vi "MP711134-12V.vi"(8 "error in (no error)":errorcluster) -> (0 "error in (out)":errorcluster)   [LabVIEW 2024, in "Multicom_MP711134-12V.lvlib"]
doc: "This template is for the Queued Message Handler design pattern.\n\nThe Event Handling Loop generates messages based on user interface actions.\n\nThe Message Handling Loop processes messages generated by the Event Handling Loop, or by other messages. The messages are string values, so new messages can be added easily to the Message Cases case structure in the Message Handling Loop. Each message cluster can also provide an optional value for Message Data, which is a variant that can be converted to whatever message-specific data is required."
uses:
  Multicom_MP711134-12V.lvlib
  controls/72-13360 UI Data.ctl
  PrivateControls/FGV_Queue_Control.ctl
  <vilib>/Instr/_visa.llb/VISA Configure Serial Port (Instr).vi
  <vilib>/Utility/error.llb/Error Cluster From Error Code.vi
  <vilib>/ErrorRing/Error Ring.xnode
  support/Message Queue/72-13360 Message Queue.lvlib
  support/User Event - Stop/72-13360 User Event - Stop.lvlib
  Launcher/Launcher_DTU.lvlib
panel:
  in  "Config":string
  in  "DUT":string
  out "RESISTANCE":string
  out "CURRENT":string
  out "VOLTAGE":string
  in  "VISA resource name":refnum<visa-resource-name>
  in  "SET_Current":dbl format="%#_4f"
  in  "SET_Voltage":dbl format="%#_4f"
  in  "Read_Res":bool
  in  "Read_Current":bool
  in  "Read_Voltage":bool
  in  "Set Current":bool
  out "Connected?":bool
  out "queue name 2":string
  out "queue name":string
  out "Display <Replace Me>":string
  in  "Output":bool
  in  "Set Voltage":bool
  in  "Exit":bool
  # "These controls have associated \"Value Changed\" events configured in the Event Structure on the diagram.\n\nReplace them (and reconfigure the Event Structure) with the controls you need for your application."
  # "This template is for the Queued Message Handler design pattern.\n\nSee the block diagram for more information on how to use this template."
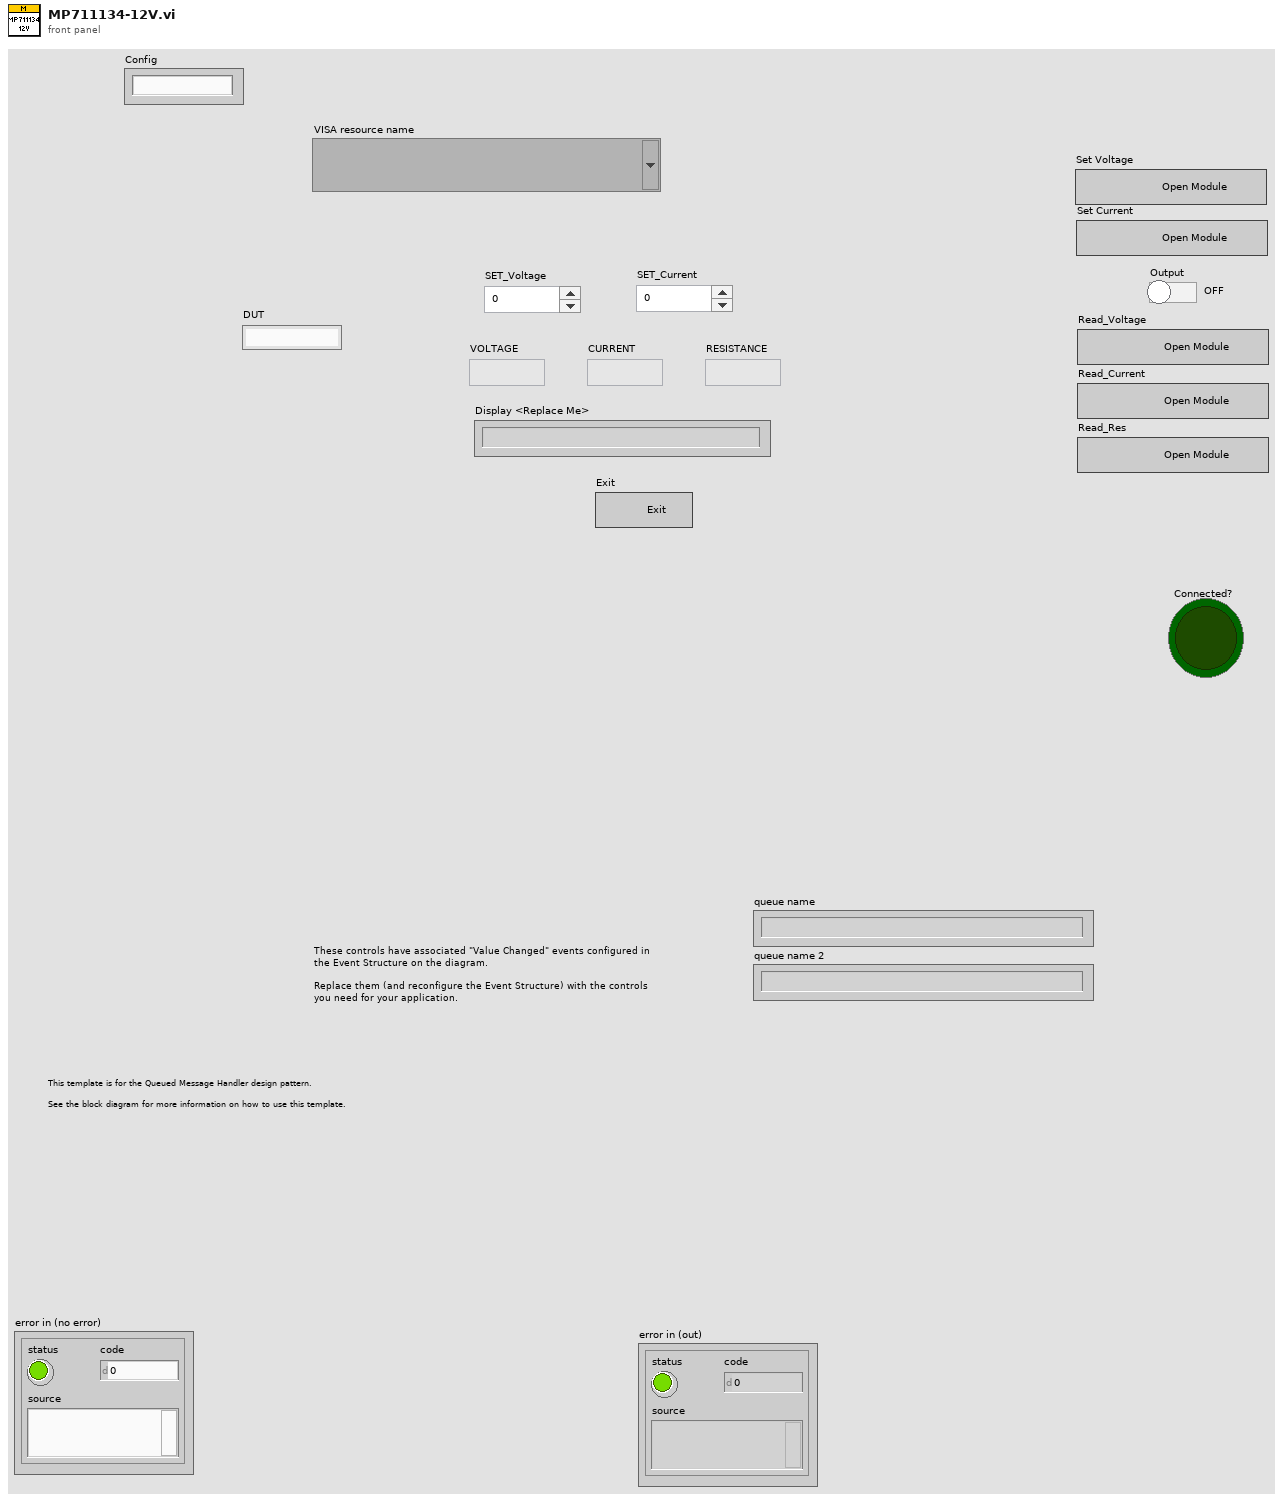
[diagram p1: front panel]
types:
  T1 = typedef "Multicom_MP711134-12V.lvlib/72-13360 UI Data.ctl" = cluster{"Boolean <Replace Me>":bool, "DUT":string, "Numeric <Replace Me>":dbl, "VISA":refnum<visa-resource-name>, "13360_Q":refnum<queue>, "notifier out":refnum<notifier>, "Config":string}
  T2 = typedef "Multicom_MP711134-12V.lvlib/FGV_Queue_Control.ctl" = enum16{"Release", "Get", "Set"}
  T3 = typedef "Multicom_MP711134-12V.lvlib/72-13360 Message Queue.lvlib/All Message Queues.ctl" = cluster{"UI":refnum<queue>, "QSM":refnum<queue>}
  T4 = cluster{"Message":string, "Message Data":variant}
  T5 = enum16{"Read", "Write", "All_sections", "All_values", "Remove key&section"}
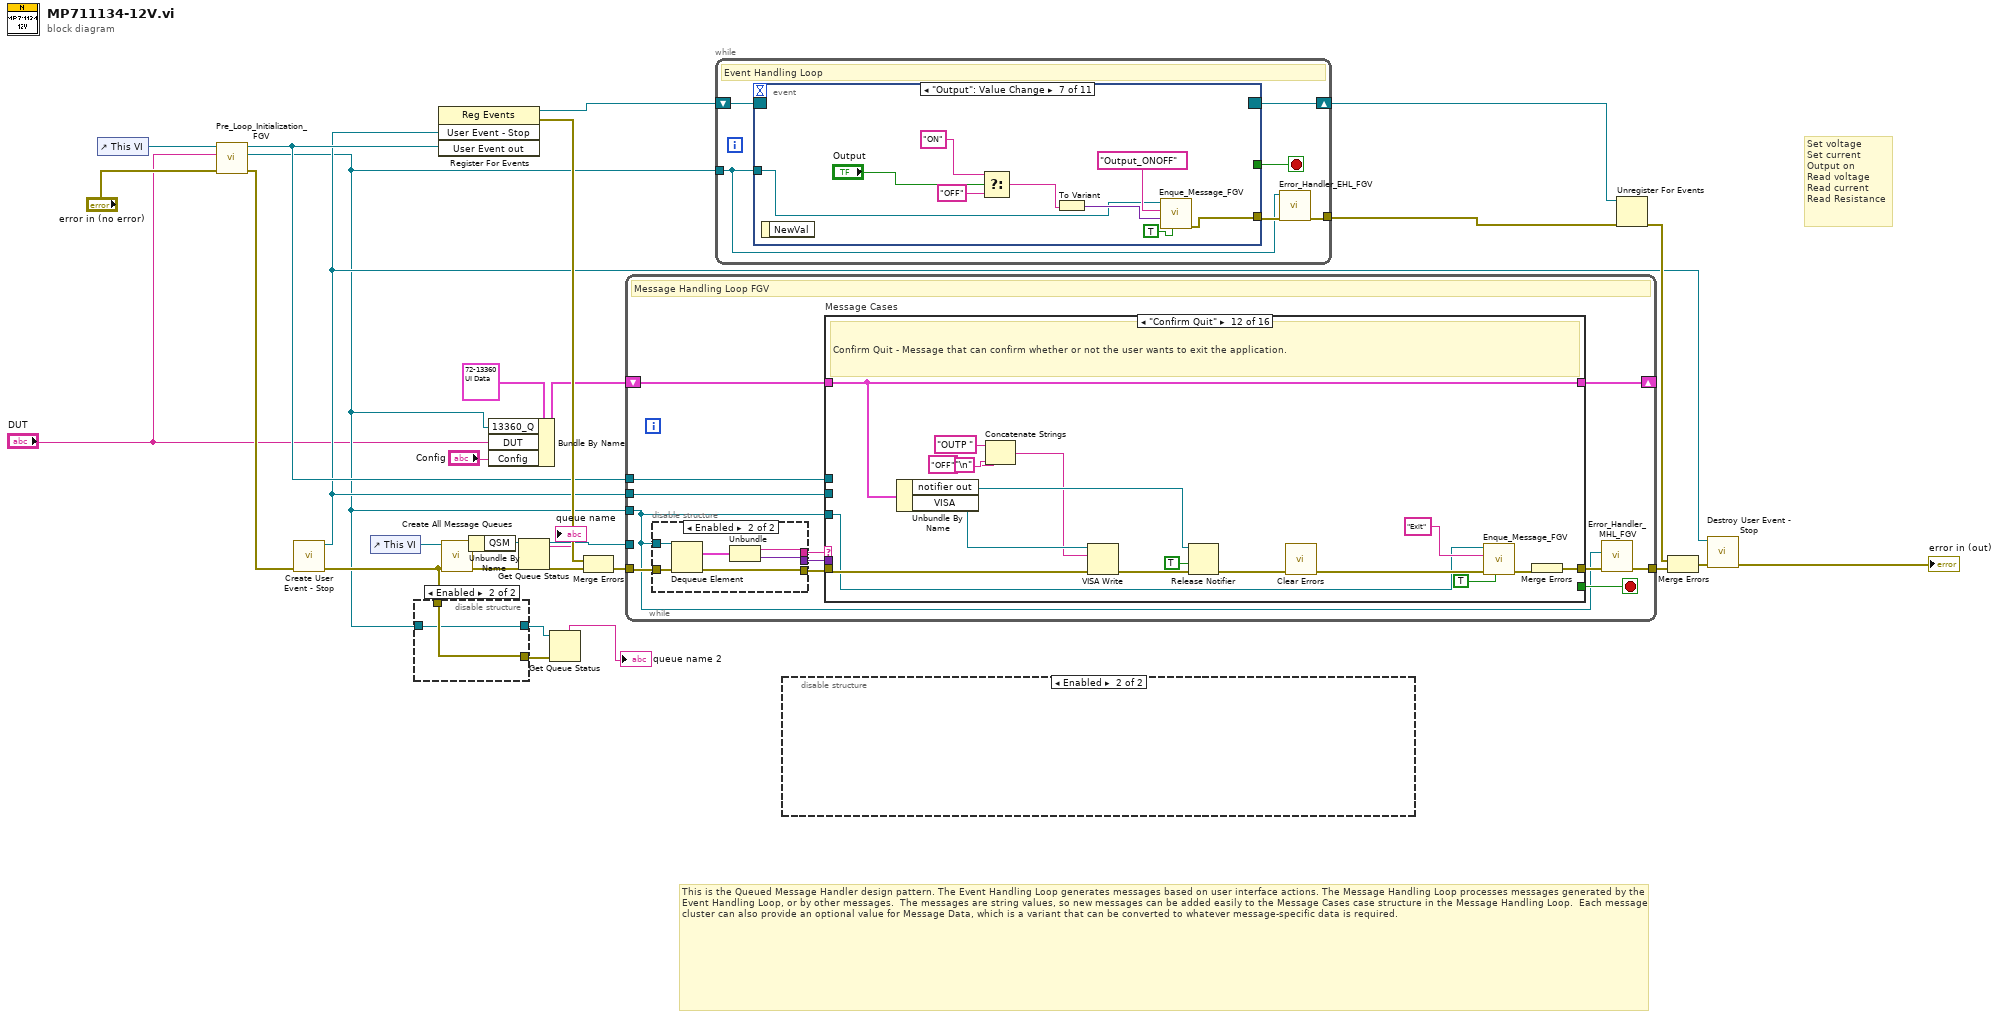
[diagram p0: block diagram]
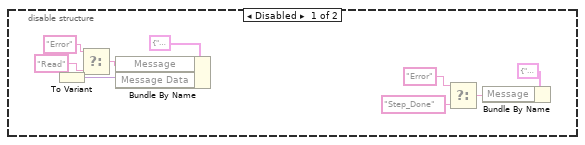
[diagram p2: hidden frame]
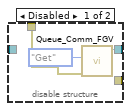
[diagram p3: hidden frame]
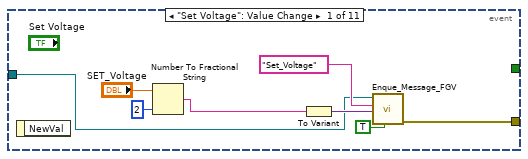
[diagram p4: hidden frame]
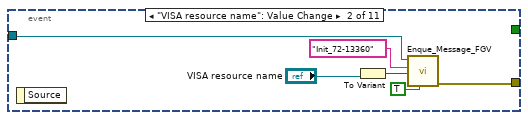
[diagram p5: hidden frame]
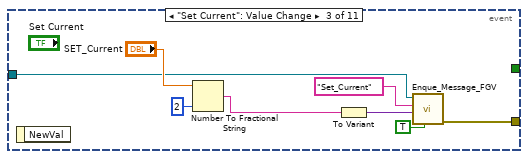
[diagram p6: hidden frame]
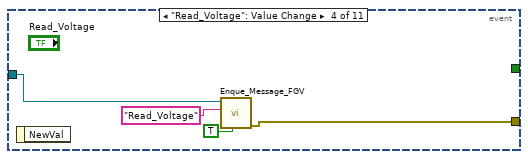
[diagram p7: hidden frame]
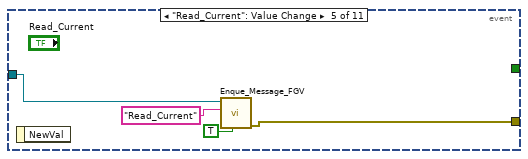
[diagram p8: hidden frame]
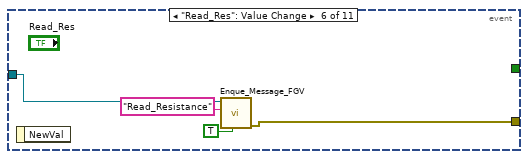
[diagram p9: hidden frame]
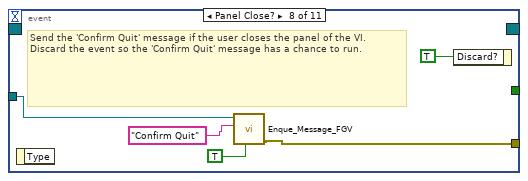
[diagram p10: hidden frame]
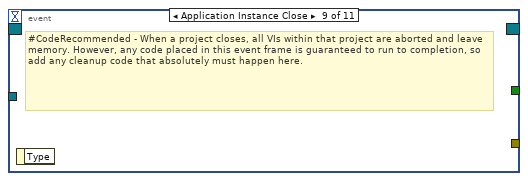
[diagram p11: hidden frame]
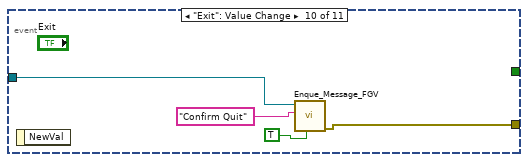
[diagram p12: hidden frame]
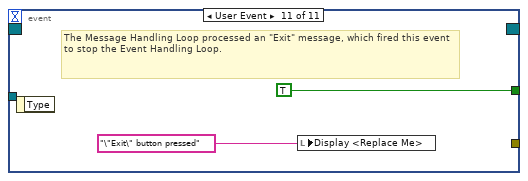
[diagram p13: hidden frame]
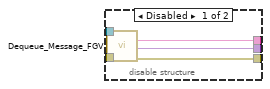
[diagram p14: hidden frame]
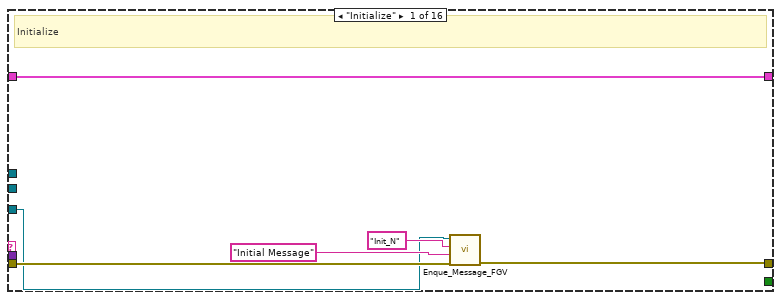
[diagram p15: hidden frame]
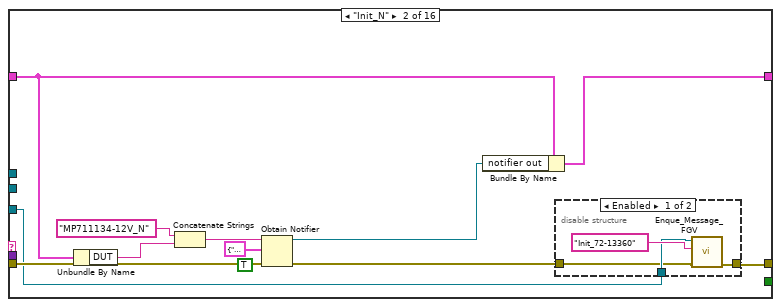
[diagram p16: hidden frame]
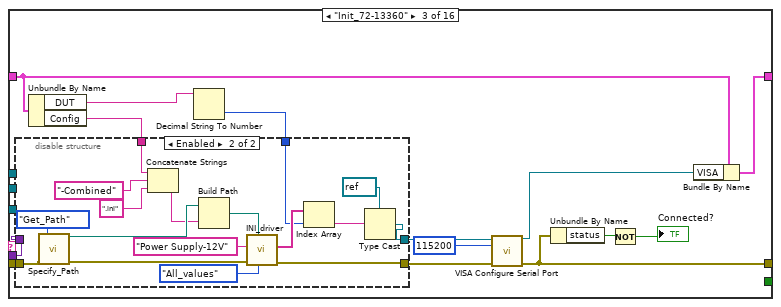
[diagram p18: hidden frame]
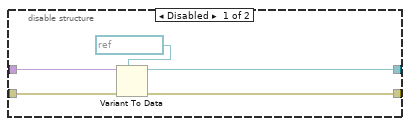
[diagram p19: hidden frame]
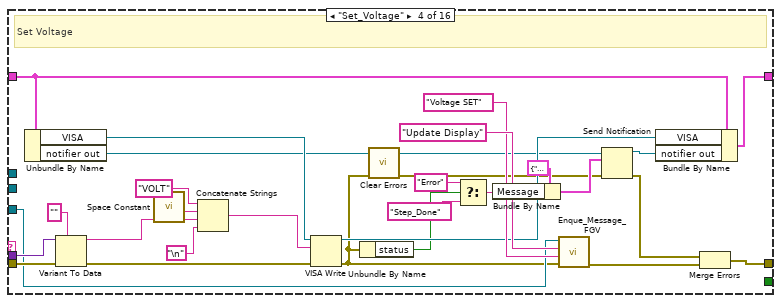
[diagram p20: hidden frame]
diagram:
  # "Set voltage\nSet current\nOutput on\nRead voltage \nRead current\nRead Resistance"
  # "This is the Queued Message Handler design pattern. The Event Handling Loop generates messages based on user interface actions. The Message Handling Loop processes messages generated by the Event Handling Loop, or by other messages.  The messages are string values, so new messages can be added easily to the Message Cases case structure in the Message Handling Loop.  Each message cluster can also provide an optional value for Message Data, which is a variant that can be converted to whatever message-specific data is required."
  n1 = control-ref of="This VI"() -> (w17:refnum<vi>)
  n2 = call "Pre_Loop_Initialization_FGV.vi"("error in (no error)"="error in (no error)", "DUT"="DUT", "VI in"=w17) -> ("error out"=w15:errorcluster, "queue out"=w3:refnum<queue>, "User Event out"=w7:refnum<user-event>)  [unwired: 6 in]
  n3 = call "Create User Event - Stop.vi"("error in (no error)"=w15) -> ("error out"=w10:errorcluster, "User Event - Stop"=w6:refnum<user-event>)  [unwired: 9 in]
  n4 = control-ref of="This VI"() -> (w13:refnum<vi>)
  n5 = disable-structure shown="Enabled" {
    disable-tunnel: w10 -> [w32 w34]
    disable-tunnel: [w30 w33] -> w9
    disable-tunnel: [_ w34] -> w5
    disable-tunnel: w3 -> [_ w33]
    frame Disabled {
      n6 = call "Queue_Comm_FGV.vi"("error in (no error)"=w32, "Enum"=FGV_Queue_Control."Get") -> ("queue Out"=w30:refnum<queue>)  [unwired: 8 in, 1 out]
    }
    frame Enabled {
    }
  }
  n7 = register-events(w6, w7) -> (reference out=w20:refnum<event-registration>, error out=w18:errorcluster)  [unwired: 2 in]
  n8 = call "Create All Message Queues.vi"("error in (no error)"=w10, "This VI"=w13) -> ("error out"=w29:errorcluster, "Message Queues out"=w28:T3)  [unwired: 8 in]
  n9 = Unbundle By Name(w28) -> ("QSM"=w26:refnum<queue>)
  n10 = Bundle By Name(cluster=T1 {"Boolean <Replace Me>"=FALSE, "DUT"="", "Numeric <Replace Me>"=0.0, "VISA"="", "13360_Q"=refnum, "notifier out"=refnum, "Config"=""} ("Data Cluster"), "13360_Q"=w3, "DUT"="DUT", "Config"="Config") -> (w4:T1)
  n11 = Get Queue Status(queue=w26) -> (queue out=w12:refnum<queue>, queue name=→"queue name":string)  [unwired: 2 in, 6 out]
  n12 = Get Queue Status(queue=w9, error in (no error)=w5) -> (queue name=→"queue name 2":string)  [unwired: 1 in, 7 out]
  n13 = Merge Errors(w18, w29) -> (w19:errorcluster)
  n14 = while {
    tunnel: w12 -> [_]
    shift-right: [w45] -> _
    shift-left: w4 -> [w46]
    tunnel: w7 -> [w43]
    tunnel: w19 -> [w42]
    tunnel: [w37] -> w27
    tunnel: w6 -> [w36]
    tunnel: w3 -> [w35]
    stop <- w44 stop-if-true
    # "Message Handling Loop FGV"
    n15 = disable-structure shown="Enabled" {
      disable-tunnel: w42 -> [w50 w56]
      disable-tunnel: [w49 w54] -> w41
      disable-tunnel: [w48 w51] -> w40
      disable-tunnel: [w47 w52] -> w39
      disable-tunnel: w35 -> [_ w55]
      frame Disabled {
        n16 = call "Dequeue_Message_FGV.vi"("error in (no error)"=w50) -> ("error out"=w49:errorcluster, "Message Data"=w48:variant, "Message"=w47:string)  [unwired: 8 in]
      }
      frame Enabled {
        n17 = Dequeue Element(queue=w55, error in (no error)=w56) -> (element=w53:T4, error out=w54:errorcluster)  [unwired: 1 in, 2 out]
        n18 = Unbundle(w53) -> ("Message"=w52:string, "Message Data"=w51:variant)
      }
    }
    n19 = case "Message Cases" shown="\"Confirm Quit\"" w39 {
      selector: w39 -> [_ _ _ _ _ _ _ _ _ _ _ _ _ _ _ w340]
      tunnel: w41 -> [w58 w74 w93 w140 w157 w200 w235 w243 w274 w281 w291 w306 w317 w320 w331 _]
      tunnel: [w61 w63 w89 w144 w169 w183 w218 w242 w258 w282 w285 w308 w314 w318 w321 w341] -> w38
      tunnel: w46 -> [w62 w72 w83 w136 w159 w198 w233 w246 w270 w283 w290 w303 w316 w319 w326 w342]
      tunnel: [w62 w67 w92 w134 w159 w196 w231 w246 w264 w283 w290 w303 w316 w319 w326 w342] -> w45
      tunnel: [_ _ _ _ _ _ _ _ _ _ _ _ _ _ TRUE _] -> w44
      tunnel: w40 -> [_ _ w85 w138 w161 _ _ _ w267 w280 w289 _ _ _ w333 _]
      tunnel: w43 -> [_ _ _ _ _ _ _ _ _ _ _ _ _ _ w334 _]
      tunnel: w36 -> [_ _ _ _ _ _ _ _ _ _ _ _ _ _ w329 _]
      tunnel: w35 -> [w57 w65 _ w128 w155 w184 w219 w241 w259 _ _ w299 _ _ w322 _]
      frame "Initialize" {
        # "Initialize"
        n20 = call "Enque_Message_FGV.vi"("error in (no error)"=w58, "Message Data"="Initial Message" ("Initial Message"), "Message"="Init_N", "queue in"=w57) -> ("error out"=w61:errorcluster)  [unwired: 7 in]
      }
      frame "Init_N" {
        n21 = Unbundle By Name(w72) -> ("DUT"=w71:string)
        n22 = Concatenate Strings("MP711134-12V_N", w71) -> (w70:string)
        n23 = Obtain Notifier(name (unnamed)=w70, notification data type=T4 {"Message"="", "Message Data"=variant} ("notification"), create if not found? (T)=TRUE, error in (no error)=w74) -> (notifier out=w66:refnum<notifier>, error out=w64:errorcluster)  [unwired: 1 out]
        n24 = Bundle By Name(cluster=w72, "notifier out"=w66) -> (w67:T1)
        n25 = disable-structure shown="Enabled" {
          disable-tunnel: w65 -> [w77 _]
          disable-tunnel: w64 -> [w76 w79]
          disable-tunnel: [w75 w79] -> w63
          frame Enabled {
            n26 = call "Enque_Message_FGV.vi"("error in (no error)"=w76, "Message"="Init_72-13360", "queue in"=w77) -> ("error out"=w75:errorcluster)  [unwired: 8 in]
          }
          frame Disabled {
          }
        }
      }
      frame "Init_72-13360" {
        n27 = Unbundle By Name(w83) -> ("DUT"=w81:string, "Config"=w82:string)
        n28 = Decimal String To Number(string=w81) -> (number=w80:i32)  [unwired: 2 in, 1 out]
        n29 = disable-structure shown="Enabled" {
          disable-tunnel: w93 -> [w98 w103]
          disable-tunnel: [w97 w101] -> w86
          disable-tunnel: w85 -> [w96 _]
          disable-tunnel: [w94 w102] -> w84
          disable-tunnel: w82 -> [_ w100]
          disable-tunnel: w80 -> [_ w99]
          frame Disabled {
            n30 = Variant To Data(error in=w98, type=refnum<visa-resource-name> "COM27" ("VISA resource name"), Variant=w96) -> (data=w94:refnum<visa-resource-name>, error out=w97:errorcluster)
          }
          frame Enabled {
            n31 = call "Specify_Path.vi"("Path_Enum"=enum16{"Find_Path", "Get_Path"}."Get_Path", "error in (no error)"=w103) -> ("Configurations"=w112:path, "error out"=w108:errorcluster)  [unwired: 6 in, 6 out]
            n32 = Concatenate Strings(w100, "-Combined" ("string"), ".ini" ("string")) -> (w111:string)
            n33 = Build Path(base path=w112, name or relative path=w111) -> (appended path=w110:path)
            n34 = call "INI_driver.vi"("Enum"=T5."All_values", "instrument file path"=w110, "error in (no error)"=w108, "Section"="Power Supply-12V") -> ("error out"=w101:errorcluster, "Values out"=w106:string[])  [unwired: 4 in, 2 out]
            n35 = Index Array(array=w106, index=w99) -> (element=w105:string)
            n36 = Type Cast(type=refnum<visa-resource-name> refnum ("VISA resource name"), x=w105) -> (*(type *) &x=w102:refnum<visa-resource-name>)
          }
        }
        n37 = call-poly "VISA Configure Serial Port"("VISA resource name"=w84, "baud rate (9600)"=u32 115200, "error in (no error)"=w86) -> ("VISA resource name out"=w90:refnum<visa-resource-name>, "error out"=w89:errorcluster)  [unwired: 11 in]
        n38 = Unbundle By Name(w89) -> ("status"=w88:bool)
        n39 = Not(x=w88) -> (.not. x?=→"Connected?":bool)
        n40 = Bundle By Name(cluster=w83, "VISA"=w90) -> (w92:T1)
      }
      frame "Set_Voltage" {
        # "Set Voltage"
        n41 = Unbundle By Name(w136) -> ("VISA"=w129:refnum<visa-resource-name>, "notifier out"=w122:refnum<notifier>)
        n42 = Variant To Data(error in=w140, type="", Variant=w138) -> (data=w131:string, error out=w139:errorcluster)
        n43 = call <vilib>:"Space Constant.vi"() -> ("String"=w116:string)
        n44 = Concatenate Strings("VOLT", w116, w131, "\n") -> (w132:string)
        n45 = VISA Write(VISA resource name=w129, write buffer=w132, error in (no error)=w139) -> (VISA resource name out=w133:refnum<visa-resource-name>, error out=w118:errorcluster)  [unwired: 1 out]
        n46 = Unbundle By Name(w118) -> ("status"=w117:bool)
        n47 = call <vilib>:"Clear Errors.vi"("error in (no error)"=w118) -> ("error out"=w119:errorcluster)  [unwired: 5 in, 1 out]
        n48 = Select(t="Error" ("f"), s=w117, f="Step_Done" ("Message")) -> (s? t:f=w125:string)
        n49 = Bundle By Name(cluster=T4 {"Message"="", "Message Data"=variant} ("notification"), "Message"=w125) -> (w121:T4)
        n50 = call "Enque_Message_FGV.vi"("error in (no error)"=w118, "Message Data"="Voltage SET" ("\"Do Something\" button pressed"), "Message"="Update Display", "queue in"=w128) -> ("error out"=w143:errorcluster)  [unwired: 7 in]
        n51 = Send Notification(notification=w121, notifier=w122, error in (no error)=w119) -> (notifier out=w123:refnum<notifier>, error out=w120:errorcluster)
        n52 = Bundle By Name(cluster=w136, "VISA"=w133, "notifier out"=w123) -> (w134:T1)
        n53 = Merge Errors(w120, w143) -> (w144:errorcluster)
      }
      frame "Set_Current" {
        # "Set current"
        n54 = Unbundle By Name(w159) -> ("notifier out"=w154:refnum<notifier>, "VISA"=w156:refnum<visa-resource-name>)
        n55 = Variant To Data(type="", Variant=w161) -> (data=w160:string)  [unwired: 1 in, 1 out]
        n56 = call <vilib>:"Space Constant.vi"() -> ("String"=w162:string)
        n57 = Concatenate Strings("CURR", w162, w160, "\n") -> (w163:string)
        n58 = VISA Write(VISA resource name=w156, write buffer=w163, error in (no error)=w157) -> (error out=w146:errorcluster)  [unwired: 2 out]
        n59 = Unbundle By Name(w146) -> ("status"=w145:bool)
        n60 = Select(t="Error" ("f"), s=w145, f="Step_Done" ("Message")) -> (s? t:f=w149:string)
        n61 = call <vilib>:"Clear Errors.vi"("error in (no error)"=w146) -> ("error out"=w153:errorcluster)  [unwired: 5 in, 1 out]
        n62 = Bundle By Name(cluster=T4 {"Message"="", "Message Data"=variant} ("notification"), "Message"=w149) -> (w147:T4)
        n63 = Send Notification(notification=w147, notifier=w154, error in (no error)=w153) -> (error out=w152:errorcluster)  [unwired: 1 out]
        n64 = call "Enque_Message_FGV.vi"("error in (no error)"=w146, "Message Data"="CURRENT SET" ("\"Do Something\" button pressed"), "Message"="Update Display", "queue in"=w155) -> ("error out"=w168:errorcluster)  [unwired: 7 in]
        n65 = Merge Errors(w152, w168) -> (w169:errorcluster)
      }
      frame "Read_Voltage" {
        # "Read Voltage"
        n66 = Unbundle By Name(w198) -> ("notifier out"=w181:refnum<notifier>, "VISA"=w197:refnum<visa-resource-name>)
        n67 = Concatenate Strings("MEAS:VOLT?", "\n") -> (w185:string)
        n68 = VISA Write(VISA resource name=w197, write buffer=w185, error in (no error)=w200) -> (VISA resource name out=w193:refnum<visa-resource-name>, error out=w194:errorcluster)  [unwired: 1 out]
        n69 = flat-sequence {
          tunnel: w194 -> [w205]
          tunnel: [w205] -> w188
          tunnel: w193 -> [w204]
          tunnel: [w204] -> w189
          frame #0 {
            n70 = Wait (ms)(milliseconds to wait=u32 500) -> ()  [unwired: 1 out]
          }
        }
        n71 = property class="Instr"(reference=w189, error in=w188) -> (reference out=w192:refnum<visa-resource-name>, error out=w191:errorcluster, "Bytes at Port"=w190:u32)
        n72 = VISA Read(VISA resource name=w192, byte count=w190, error in (no error)=w191) -> (VISA resource name out=w195:refnum<visa-resource-name>, read buffer=w174:string, error out=w172:errorcluster)  [unwired: 1 out]
        "VOLTAGE" <- w174
        n73 = To Variant(anything=w174) -> (Variant=w177:variant)
        n74 = Unbundle By Name(w172) -> ("status"=w171:bool)
        n75 = Select(t="Error" ("f"), s=w171, f="Read" ("Message")) -> (s? t:f=w180:string)
        n76 = Bundle By Name(cluster=T4 {"Message"="", "Message Data"=variant} ("notification"), "Message"=w180, "Message Data"=w177) -> (w175:T4)
        n77 = call <vilib>:"Clear Errors.vi"("error in (no error)"=w172) -> ("error out"=w173:errorcluster)  [unwired: 5 in, 1 out]
        n78 = Send Notification(notification=w175, notifier=w181, error in (no error)=w173) -> (notifier out=w182:refnum<notifier>, error out=w170:errorcluster)
        n79 = Bundle By Name(cluster=w198, "VISA"=w195, "notifier out"=w182) -> (w196:T1)
        n80 = call "Enque_Message_FGV.vi"("error in (no error)"=w172, "Message Data"="Read Voltage" ("\"Do Something\" button pressed"), "Message"="Update Display", "queue in"=w184) -> ("error out"=w199:errorcluster)  [unwired: 7 in]
        n81 = Merge Errors(w170, w199) -> (w183:errorcluster)
      }
      frame "Read_Current" {
        # "Read Voltage"
        n82 = Unbundle By Name(w233) -> ("notifier out"=w206:refnum<notifier>, "VISA"=w232:refnum<visa-resource-name>)
        n83 = Concatenate Strings("MEAS:CURR?", "\n") -> (w220:string)
        n84 = VISA Write(VISA resource name=w232, write buffer=w220, error in (no error)=w235) -> (VISA resource name out=w228:refnum<visa-resource-name>, error out=w229:errorcluster)  [unwired: 1 out]
        n85 = flat-sequence {
          tunnel: w229 -> [w240]
          tunnel: [w240] -> w223
          tunnel: w228 -> [w239]
          tunnel: [w239] -> w224
          frame #0 {
            n86 = Wait (ms)(milliseconds to wait=u32 500) -> ()  [unwired: 1 out]
          }
        }
        n87 = property class="Instr"(reference=w224, error in=w223) -> (reference out=w227:refnum<visa-resource-name>, error out=w226:errorcluster, "Bytes at Port"=w225:u32)
        n88 = VISA Read(VISA resource name=w227, byte count=w225, error in (no error)=w226) -> (VISA resource name out=w230:refnum<visa-resource-name>, read buffer=w210:string, error out=w209:errorcluster)  [unwired: 1 out]
        "CURRENT" <- w210
        n89 = To Variant(anything=w210) -> (Variant=w213:variant)
        n90 = Unbundle By Name(w209) -> ("status"=w208:bool)
        n91 = Select(t="Error" ("f"), s=w208, f="Read" ("Message")) -> (s? t:f=w216:string)
        n92 = Bundle By Name(cluster=T4 {"Message"="", "Message Data"=variant} ("notification"), "Message"=w216, "Message Data"=w213) -> (w211:T4)
        n93 = call <vilib>:"Clear Errors.vi"("error in (no error)"=w209) -> ("error out"=w217:errorcluster)  [unwired: 5 in, 1 out]
        n94 = Send Notification(notification=w211, notifier=w206, error in (no error)=w217) -> (error out=w207:errorcluster)  [unwired: 1 out]
        n95 = call "Enque_Message_FGV.vi"("error in (no error)"=w209, "Message Data"="Read CURRENT" ("\"Do Something\" button pressed"), "Message"="Update Display", "queue in"=w219) -> ("error out"=w234:errorcluster)  [unwired: 7 in]
        n96 = Bundle By Name(cluster=w233, "VISA"=w230) -> (w231:T1)
        n97 = Merge Errors(w207, w234) -> (w218:errorcluster)
      }
      frame "Read_Resistance" {
        # "Set Resistance"
        n98 = call "Enque_Message_FGV.vi"("error in (no error)"=w243, "Message Data"="\"Do Something\" button pressed" ("\"Do Something\" button pressed"), "Message"="Update Display", "queue in"=w241) -> ("error out"=w242:errorcluster)  [unwired: 7 in]
      }
      frame "Output_ONOFF" {
        # "Something Else - Replace this message with functionality for your own application."
        n99 = Unbundle By Name(w270) -> ("notifier out"=w254:refnum<notifier>, "VISA"=w269:refnum<visa-resource-name>)
        n100 = Variant To Data(error in=w274, type="", Variant=w267) -> (data=w265:string, error out=w268:errorcluster)
        n101 = Concatenate Strings("OUTP " ("string"), w265, "\n") -> (w262:string)
        n102 = VISA Write(VISA resource name=w269, write buffer=w262, error in (no error)=w268) -> (VISA resource name out=w263:refnum<visa-resource-name>, error out=w255:errorcluster)  [unwired: 1 out]
        n103 = Unbundle By Name(w255) -> ("status"=w249:bool)
        n104 = Select(t="Error" ("f"), s=w249, f="Step_Done" ("Message")) -> (s? t:f=w251:string)
        n105 = call <vilib>:"Clear Errors.vi"("error in (no error)"=w255) -> ("error out"=w256:errorcluster)  [unwired: 5 in, 1 out]
        n106 = Bundle By Name(cluster=T4 {"Message"="", "Message Data"=variant} ("notification"), "Message"=w251) -> (w248:T4)
        n107 = Send Notification(notification=w248, notifier=w254, error in (no error)=w256) -> (notifier out=w247:refnum<notifier>, error out=w257:errorcluster)
        n108 = call <vilib>:"Space Constant.vi"() -> ("String"=w271:string)
        n109 = Concatenate Strings("OUTPUT" ("\"Do Something Else\" button pressed"), w271, w265) -> (w272:string)
        n110 = Bundle By Name(cluster=w270, "VISA"=w263, "notifier out"=w247) -> (w264:T1)
        n111 = call "Enque_Message_FGV.vi"("error in (no error)"=w255, "Message Data"=w272, "Message"="Update Display", "queue in"=w259) -> ("error out"=w273:errorcluster)  [unwired: 7 in]
        n112 = Merge Errors(w257, w273) -> (w258:errorcluster)
      }
      frame "Update Display" {
        # "#CodeRecommended - If you wish to decouple the Message Handling Loop from your user interface, consider creating User Events (like the \"Stop\" event in this VI) to message the Event Handling Loop whenever the user interface needs updating."
        # "Update Display - Convert the message data to a string to display in the Data Display indicator."
        n113 = Variant To Data(error in=w281, type="", Variant=w280) -> (data=→"Display <Replace Me>":string, error out=w278:errorcluster)
        n114 = Merge Errors(w278) -> (w282:errorcluster)
      }
      frame "Error" {
        # "Error - Display an error dialog. This message is sent by the \"Error Handler\" VIs at the end of other loops in this application."
        n115 = Variant To Data(error in=w291, type=errorcluster {"status"=FALSE, "code"=0, "source"=""} ("error constant"), Variant=w289) -> (data=w287:errorcluster, error out=w286:errorcluster)
        n116 = call <vilib>:"Simple Error Handler.vi"("error in (no error)"=w287) -> ()  [unwired: 4 in, 5 out]
        n117 = call <vilib>:"Clear Errors.vi"("error in (no error)"=w286) -> ("error out"=w284:errorcluster)  [unwired: 5 in, 1 out]
        n118 = Merge Errors(w284) -> (w285:errorcluster)
      }
      frame "Confirm Quit" {
        # "Confirm Quit - Message that can confirm whether or not the user wants to exit the application."
        n119 = Unbundle By Name(w303) -> ("notifier out"=w297:refnum<notifier>, "VISA"=w301:refnum<visa-resource-name>)
        n120 = Concatenate Strings("OUTP " ("string"), "OFF" ("string"), "\n") -> (w292:string)
        n121 = VISA Write(VISA resource name=w301, write buffer=w292, error in (no error)=w306) -> (error out=w302:errorcluster)  [unwired: 2 out]
        n122 = Release Notifier(notifier=w297, force destroy? (F)=TRUE, error in (no error)=w302) -> (error out=w298:errorcluster)  [unwired: 2 out]
        n123 = call <vilib>:"Clear Errors.vi"("error in (no error)"=w298) -> ("error out"=w300:errorcluster)  [unwired: 5 in, 1 out]
        n124 = call "Enque_Message_FGV.vi"("Priority"=TRUE ("Priority Message? (F)"), "error in (no error)"=w300, "Message"="Exit", "queue in"=w299) -> ("error out"=w307:errorcluster)  [unwired: 7 in]
        n125 = Merge Errors(w307) -> (w308:errorcluster)
      }
      frame "Reset" {
        (unwired) TRUE ("force destroy? (F)")
        # "Confirm Quit - Message that can confirm whether or not the user wants to exit the application."
        n126 = Unbundle By Name(w316) -> ("VISA"=w315:refnum<visa-resource-name>)
        n127 = Concatenate Strings("OUTP " ("string"), "OFF" ("string"), "\n") -> (w311:string)
        n128 = VISA Write(VISA resource name=w315, write buffer=w311, error in (no error)=w317) -> (error out=w313:errorcluster)  [unwired: 2 out]
        n129 = call <vilib>:"Clear Errors.vi"("error in (no error)"=w313) -> ("error out"=w314:errorcluster)  [unwired: 5 in, 1 out]
      }
      frame "---Copy This Frame---" {
        # "Duplicate this frame when creating new messages.  Change this comment in the duplicated frame to describe this message."
        n130 = Merge Errors(w320) -> (w318:errorcluster)
      }
      frame "Exit" {
        # "Stop the VI"
        # "Release the message queue reference"
        # "Exit - Exit the application."
        n131 = disable-structure shown="Disabled" {
          disable-tunnel: w333 -> [w337 _]
          frame Disabled {
            n132 = Variant To Data(type=errorcluster {"status"=FALSE, "code"=0, "source"=""} ("error constant"), Variant=w337) -> (data=w338:errorcluster)  [unwired: 1 in, 1 out]
            n133 = call <vilib>:"Simple Error Handler.vi"("error in (no error)"=w338) -> ()  [unwired: 4 in, 5 out]
          }
          frame Enabled {
          }
        }
        n134 = Unbundle By Name(w326) -> ("VISA"=w325:refnum<visa-resource-name>)
        n135 = VISA Close(VISA resource name=w325) -> (error out=w324:errorcluster)  [unwired: 1 in]
        n136 = call "Queue_Comm_FGV.vi"("error in (no error)"=w331, "Enum"=FGV_Queue_Control."Release", "queue in"=w322) -> ("error Out"=w330:errorcluster)  [unwired: 7 in, 1 out]
        n137 = call "Fire User Event - Stop.vi"("User Event - Stop"=w329) -> ("error out"=w327:errorcluster)  [unwired: 10 in]
        n138 = call <vilib>:"Clear Errors.vi"("error in (no error)"=w324) -> ("error out"=w323:errorcluster)  [unwired: 5 in, 1 out]
        n139 = call "Fire User Event - Stop.vi"("User Event - Stop"=w334) -> ("error out"=w328:errorcluster)  [unwired: 10 in]
        n140 = Merge Errors(w323, w328, w327, w330) -> (w335:errorcluster)
        n141 = call <vilib>:"Clear Errors.vi"("error in (no error)"=w335) -> ("error out"=w321:errorcluster)  [unwired: 5 in, 1 out]
      }
      frame Default {
        # "'Default' case only runs if there is a message that isn't defined in any of the other cases.  Output a programming error."
        n142 = xnode "Error Ring"("parameter 0"=w340) -> ("error out"=w341:errorcluster)
      }
    }
    n143 = call "Error_Handler_MHL_FGV.vi"("error in (no error)"=w38, "queue in"=w35) -> ("error Out"=w37:errorcluster)  [unwired: 9 in]
  }
  n144 = while {
    shift-right: [w354] -> w23
    shift-left: w20 -> [w355]
    tunnel: [w351] -> w21
    tunnel: w3 -> [w350]
    stop <- w353 stop-if-true
    # "Event Handling Loop"
    n145 = event shown="[6] \"Output\": Value Change" {
      selector: w355 -> [_ _ _ _ _ _ _ _ _ _ _]
      dyn-events: [_ _ _ _ _ _ _ _ _ _ _] -> w354
      timeout: _ -> [_ _ _ _ _ _ _ _ _ _ _]
      tunnel: [_ _ _ _ _ _ _ _ _ _ TRUE ("Discard?")] -> w353
      tunnel: [w362 w367 w376 w380 w384 w388 w396 w402 _ w407 _] -> w352
      tunnel: w350 -> [w356 w364 w370 w378 w382 w386 w390 w399 _ w404 _]
      event "Set Voltage": Value Change {
        n146 = event-data() -> ()  [unwired: 1 in, 1 out]
        n147 = Number To Fractional String(number="SET_Voltage", precision (6)=i16 2) -> (F-format string=w359:string)  [unwired: 2 in]
        n148 = To Variant(anything=w359) -> (Variant=w357:variant)
        n149 = call "Enque_Message_FGV.vi"("Priority"=TRUE ("Priority Message? (F)"), "Message Data"=w357, "Message"="Set_Voltage", "queue in"=w356) -> ("error out"=w362:errorcluster)  [unwired: 7 in]
      }
      event "VISA resource name": Value Change {
        n150 = event-data() -> ()  [unwired: 1 in, 1 out]
        n151 = To Variant(anything="VISA resource name") -> (Variant=w366:variant)
        n152 = call "Enque_Message_FGV.vi"("Priority"=TRUE ("Priority Message? (F)"), "Message Data"=w366, "Message"="Init_72-13360", "queue in"=w364) -> ("error out"=w367:errorcluster)  [unwired: 7 in]
      }
      event "Set Current": Value Change {
        n153 = event-data() -> ()  [unwired: 1 in, 1 out]
        n154 = Number To Fractional String(number="SET_Current", precision (6)=i16 2) -> (F-format string=w373:string)  [unwired: 2 in]
        n155 = To Variant(anything=w373) -> (Variant=w372:variant)
        n156 = call "Enque_Message_FGV.vi"("Priority"=TRUE ("Priority Message? (F)"), "Message Data"=w372, "Message"="Set_Current", "queue in"=w370) -> ("error out"=w376:errorcluster)  [unwired: 7 in]
      }
      event "Read_Voltage": Value Change {
        n157 = event-data() -> ()  [unwired: 1 in, 1 out]
        n158 = call "Enque_Message_FGV.vi"("Priority"=TRUE ("Priority Message? (F)"), "Message"="Read_Voltage", "queue in"=w378) -> ("error out"=w380:errorcluster)  [unwired: 8 in]
      }
      event "Read_Current": Value Change {
        n159 = event-data() -> ()  [unwired: 1 in, 1 out]
        n160 = call "Enque_Message_FGV.vi"("Priority"=TRUE ("Priority Message? (F)"), "Message"="Read_Current", "queue in"=w382) -> ("error out"=w384:errorcluster)  [unwired: 8 in]
      }
      event "Read_Res": Value Change {
        n161 = event-data() -> ()  [unwired: 1 in, 1 out]
        n162 = call "Enque_Message_FGV.vi"("Priority"=TRUE ("Priority Message? (F)"), "Message"="Read_Resistance", "queue in"=w386) -> ("error out"=w388:errorcluster)  [unwired: 8 in]
      }
      event "Output": Value Change {
        n163 = event-data() -> ()  [unwired: 1 in, 1 out]
        n164 = Select(t="ON", s="Output", f="OFF") -> (s? t:f=w392:string)
        n165 = To Variant(anything=w392) -> (Variant=w391:variant)
        n166 = call "Enque_Message_FGV.vi"("Priority"=TRUE ("Priority Message? (F)"), "Message Data"=w391, "Message"="Output_ONOFF", "queue in"=w390) -> ("error out"=w396:errorcluster)  [unwired: 7 in]
      }
      event Panel Close? {
        # "Send the 'Confirm Quit' message if the user closes the panel of the VI. Discard the event so the 'Confirm Quit' message has a chance to run."
        n167 = event-data() -> ()  [unwired: 1 in, 1 out]
        n168 = call "Enque_Message_FGV.vi"("Priority"=TRUE ("Priority Message? (F)"), "Message"="Confirm Quit", "queue in"=w399) -> ("error out"=w402:errorcluster)  [unwired: 8 in]
        n169 = event-data("Discard?"=TRUE) -> ()  [unwired: 1 in, 1 out]
      }
      event Application Instance Close {
        # "#CodeRecommended - When a project closes, all VIs within that project are aborted and leave memory. However, any code placed in this event frame is guaranteed to run to completion, so add any cleanup code that absolutely must happen here."
        n170 = event-data() -> ()  [unwired: 1 in, 1 out]
      }
      event "Exit": Value Change {
        n171 = event-data() -> ()  [unwired: 1 in, 1 out]
        n172 = call "Enque_Message_FGV.vi"("Priority"=TRUE ("Priority Message? (F)"), "Message"="Confirm Quit", "queue in"=w404) -> ("error out"=w407:errorcluster)  [unwired: 8 in]
      }
      event User Event {
        # "The Message Handling Loop processed an \"Exit\" message, which fired this event to stop the Event Handling Loop."
        n173 = event-data() -> ()  [unwired: 1 in, 1 out]
        n174 = local write "Display <Replace Me>"("\"Exit\" button pressed" ("VI Stopped")) -> ()
      }
    }
    n175 = call "Error_Handler_EHL_FGV.vi"("error in (no error)"=w352, "queue in"=w350) -> ("error Out"=w351:errorcluster)  [unwired: 9 in]
  }
  n176 = disable-structure shown="Enabled" {
    frame Disabled {
      n177 = To Variant() -> (Variant=w417:variant)  [unwired: 1 in]
      n178 = Select(t="Error" ("f"), f="Read" ("Message")) -> (s? t:f=w412:string)  [unwired: 1 in]
      n179 = Bundle By Name(cluster=T4 {"Message"="", "Message Data"=variant} ("notification"), "Message"=w412, "Message Data"=w417) -> ()  [unwired: 1 out]
      n180 = Select(t="Error" ("f"), f="Step_Done" ("Message")) -> (s? t:f=w415:string)  [unwired: 1 in]
      n181 = Bundle By Name(cluster=T4 {"Message"="", "Message Data"=variant} ("notification"), "Message"=w415) -> ()  [unwired: 1 out]
    }
    frame Enabled {
    }
  }
  n182 = Unregister For Events(event registration refnum=w23, error in=w21) -> (error out=w24:errorcluster)
  n183 = Merge Errors(w24, w27) -> (w25:errorcluster)
  n184 = call "Destroy User Event - Stop.vi"("error in (no error)"=w25, "User Event - Stop"=w6) -> ("error out"=→"error in (out)":errorcluster)  [unwired: 9 in]
